vi "Load Pin Map to Sessions.vi"(8 "error in":errorcluster, 11 "sequence context":refnum<k7>) -> (0 "error out":errorcluster)   [LabVIEW 2020, in "NIDigitalSPI.lvlib"]
uses:
  NIDigitalSPI.lvlib
  <vilib>/MeasurementLink/MeasurementLink Session Management/Session Reservation/Initialize and Close Session Behavior.ctl
  <vilib>/MeasurementLink/MeasurementLink niDigital/Create Sessions - NSess.vi
  <vilib>/MeasurementLink/MeasurementLink TestStand Integration/MeasurementLink TestStand Integration.lvlib
  <vilib>/MeasurementLink/MeasurementLink Session Management/Session Reservation/Session Reservation.lvclass
  <vilib>/MeasurementLink/MeasurementLink niDigital/MeasurementLink niDigital.lvlib
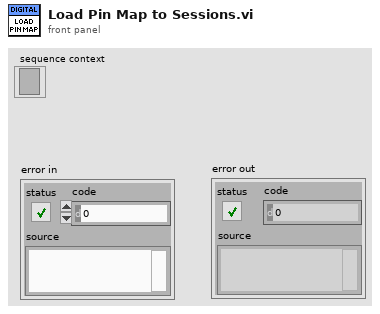
[diagram p1: front panel]
types:
  T1 = typedef "MeasurementLink Session Management.lvlib/Session Reservation.lvclass/Initialize and Close Session Behavior.ctl" = enum16{"Auto", "Initialize and Close", "Attach and Detach", "Initialize and Detach", "Attach and Close"}
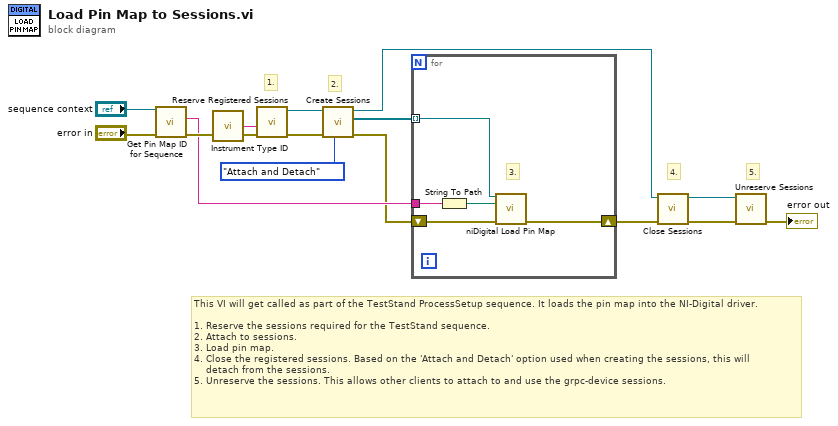
[diagram p0: block diagram]
diagram:
  # "4."
  # "5."
  # "2."
  # "1."
  # "This VI will get called as part of the TestStand ProcessSetup sequence. It loads the pin map into the NI-Digital driver.\n\n1. Reserve the sessions required for the TestStand sequence.\n2. Attach to sessions.\n3. Load pin map.\n4. Close the registered sessions. Based on the 'Attach and Detach' option used when creating the sessions, this will\n    detach from the sessions.\n5. Unreserve the sessions. This allows other clients to attach to and use the grpc-device sessions."
  n1 = call <vilib>:"Get Pin Map ID for Sequence.vi"("error in"="error in", "sequence context in"="sequence context") -> ("error out"=w11:errorcluster, "pin map id"=w10:string)  [unwired: 7 in, 1 out]
  n2 = call <vilib>:"Instrument Type ID.vi"() -> ("instrument type id"=w6:string)  [unwired: 5 in]
  n3 = call <vilib>:"Reserve Registered Sessions.vi"("error in (no error)"=w11, "instrument type id"=w6) -> ("error out"=w13:errorcluster, "session reservation out"=w12:refnum<class "Session Reservation.lvclass">)  [unwired: 8 in]
  n4 = call-poly <vilib>:"Create Sessions.vi"("initialize and close session behavior"=Initialize_and_Close_Session_Behavior."Attach and Detach", "error in"=w13, "session reservation in"=w12) -> ("error out"=w8:errorcluster, "sessions"=w9:refnum<k15>[], "session reservation out"=w1:refnum<class "Session Reservation.lvclass">)  [unwired: 5 in, 1 out]
  n5 = for {
    shift-right: [w16] -> w4
    shift-left: w8 -> [w17]
    tunnel: w10 -> [w19]
    tunnel: w9 -> [w18] mode=indexing
    # "3."
    n6 = String To Path(string=w19) -> (path=w20:path)
    n7 = call <instrlib>:"niDigital Load Pin Map.vi"("instrument handle"=w18, "pin map file"=w20, "error in"=w17) -> ("error out"=w16:errorcluster)  [unwired: 11 in, 1 out]
  }
  n8 = call <vilib>:"Close Sessions.vi"("error in"=w4, "session reservation in"=w1) -> ("error out"=w3:errorcluster, "session reservation out"=w2:refnum<class "Session Reservation.lvclass">)  [unwired: 8 in]
  n9 = call <vilib>:"Unreserve Sessions.vi"("error in"=w3, "session reservation in"=w2) -> ("error out"=→"error out":errorcluster)  [unwired: 9 in]
